vi "PH_Image_Common.Overlay Line.vi"(0 "Image":T1, 1 "Start x":i32, 2 "End x":i32, 3 "Start y":i32, 4 "End y":i32, 5 "error in (no error)":errorcluster, 9 "Color (red)":u32(colorbox)=16711680) -> (14 "Image Out":T1, 19 "error out":errorcluster)   [LabVIEW 2014, in "PH_Image_Common.lvlib"]
doc: "This VI overlays a line to an image"
uses:
  <vilib>/vision/Image Controls.llb/IMAQ Image.ctl
  PH_Image_Common.lvlib
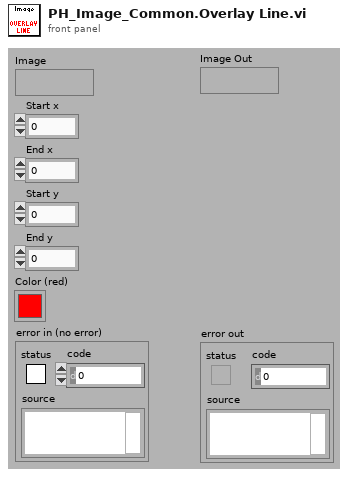
[diagram p1: front panel]
types:
  T1 = typedef "IMAQ Image.ctl" = refnum<image>
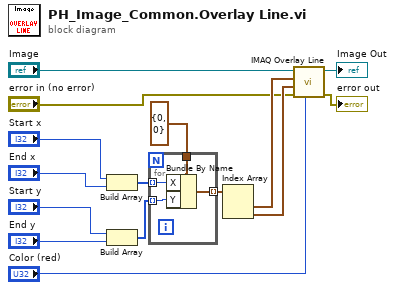
[diagram p0: block diagram]
diagram:
  n1 = Build Array("Start x", "End x") -> (w11:i32[])
  n2 = Build Array("Start y", "End y") -> (w15:i32[])
  n3 = for {
    tunnel: cluster{"X":i32, "Y":i32} {"X"=0, "Y"=0} ("Start Point") -> [w19]
    tunnel: w11 -> [w18] mode=indexing
    tunnel: [w17] -> w7 mode=indexing
    tunnel: w15 -> [w16] mode=indexing
    n4 = Bundle By Name(cluster=w19, "X"=w18, "Y"=w16) -> (w17:cluster{"X":i32, "Y":i32})
  }
  n5 = Index Array(array=w7) -> (element #1=w8:cluster{"X":i32, "Y":i32}, element #2=w9:cluster{"X":i32, "Y":i32})  [unwired: 2 in]
  n6 = call "IMAQ Overlay Line"("Color"="Color (red)", "error in (no error)"="error in (no error)", "End Point"=w9, "Start Point"=w8, "Image"="Image") -> ("error out"=→"error out":errorcluster, "Image Out"=→"Image Out":T1)  [unwired: 5 in]
